vi "CRYFlatten Acquisition.vi"(11 "Acquisition":T1={"Mode"=1, "Name"="", "use ch name"=FALSE, "Record Time"=10.0, "hide rec"=FALSE, "hide play"=FALSE, "rec delay"=0.0, "rec pad"=0.0, "dcc units"=0, "sine gen setting"="", "scope_fft setting"="", "voltmeter setting"="", "rta setting"="", "trig offset(sec)"=0.0, "triggered  record"=FALSE, "trig level"=0.0, "trig unit"=0, "trig slop"=FALSE, "trig timeout(sec)"=0.0, "add record"=FALSE, "EQ"=FALSE, "record table"=[], "play table"=[], "trig channel"="", "Help"=""} {"trig timeout(sec)" format="%.2f"; "trig level" format="%.2f"; "trig offset(sec)" format="%.2f"; "rec delay" format="%.2f"; "rec pad" format="%.2f"; "Record Time" format="%.2f"}) -> (3 "Acquisition flattened":string)   [LabVIEW 2013]
uses:
  Typedef Control/CRYAcquisition Cluster.ctl
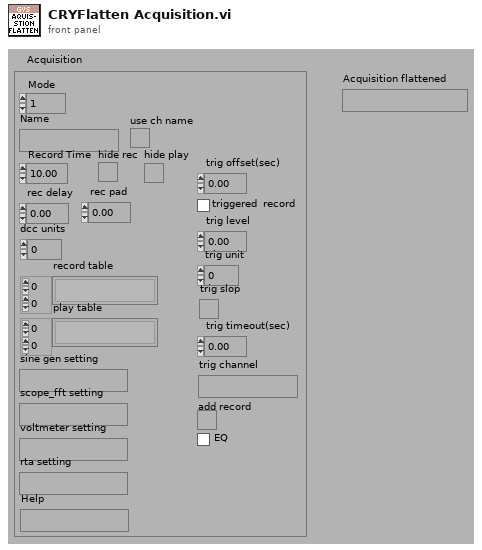
[diagram p1: front panel]
types:
  T1 = typedef "CRYAcquisition Cluster.ctl" = cluster{"Mode":u16, "Name":string, "use ch name":bool, "Record Time":dbl, "hide rec":bool, "hide play":bool, "rec delay":dbl, "rec pad":dbl, "dcc units":i8, "sine gen setting":string, "scope_fft setting":string, "voltmeter setting":string, "rta setting":string, "trig offset(sec)":dbl, "triggered  record":bool, "trig level":dbl, "trig unit":u8, "trig slop":bool, "trig timeout(sec)":dbl, "add record":bool, "EQ":bool, "record table":string[][], "play table":string[][], "trig channel":string, "Help":string}
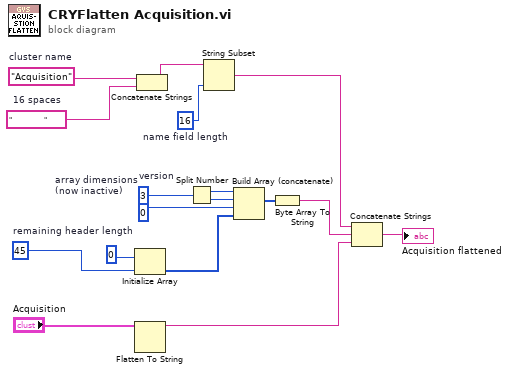
[diagram p0: block diagram]
diagram:
  w4 = u8 0  # array dimensions (now inactive)
  w7 = 16  # name field length
  w8 = "                "  # 16 spaces
  w9 = "Acquisition"  # cluster name
  w13 = 45  # remaining header length
  w17 = u16 3  # version
  n1 = Initialize Array(u8 0, w13) -> (w10:u8[])
  n2 = Flatten To String(anything="Acquisition") -> (data string=w3:string)  [unwired: 1 in, 4 out]
  n3 = Concatenate Strings(w9, w8) -> (w6:string)
  n4 = Split Number(x=w17) -> (hi(x)=w16:u8, lo(x)=w15:u8)
  n5 = String Subset(string=w6, length (rest)=w7) -> (substring=w5:string)  [unwired: 1 out]
  n6 = Build Array (concatenate)(w16, w15, w4, w10) -> (w12:u8[])
  n7 = Byte Array To String(unsigned byte array=w12) -> (string=w11:string)
  n8 = Concatenate Strings(w5, w11, w3) -> (→"Acquisition flattened":string)
